vi "Configure Trigger.vi"(8 "error in":errorcluster, 11 "DAQmx Base CFG in":refnum<class "DAQmx Base CFG.lvclass">) -> (0 "error out":errorcluster, 3 "DAQmx Base CFG out":refnum<class "DAQmx Base CFG.lvclass">)   [LabVIEW 2024, in "DAQmx Base CFG.lvclass"]
uses:
  DAQmx Base CFG.lvclass
  Configurations/CFG Base/CFG Base.lvclass/CFG Base.ctl
  <vilib>/JDP Science/JSONtext/Find Item.vi
  <vilib>/JDP Science/JSONtext/Next JSON Value.vi
  <vilib>/JDP Science/JSONtext/String Subset.vi
  <vilib>/JDP Science/JSONtext/Parsing/Advance past next JSON Value (inlined COPY).vi
  <vilib>/JDP Science/JSONtext/Parsing/Advance past whitespace.vi
  <vilib>/JDP Science/JSONtext/Parsing/Advance past String.vi
  <vilib>/JDP Science/JSONtext/Parsing/Advance past Number.vi
  <vilib>/JDP Science/JSONtext/Parsing/Advance past Line Ending.vi
  <vilib>/JDP Science/JSONtext/Parsing/Parse Full Path or Item Name.vi
  <vilib>/JDP Science/JSONtext/Parsing/Advance past Array.vi
  <vilib>/JDP Science/JSONtext/Parsing/Advance past Object.vi
  <vilib>/JDP Science/JSONtext/support/Error Cluster From Code.vi
  <vilib>/JDP Science/JSONtext/Offset/Find Item Locations by Path.vi
  <vilib>/JDP Science/JSONtext/JSON text to Variant.vi
  <vilib>/JDP Science/JSONtext/LVClass Serializer/JSONtext LVClass Serializer.lvclass
  DAQmx Base CFG.lvclass/DAQmx Base CFG.ctl
  D:/git/HAL/HAL/Configurations/CFG JSON/CFG JSON.lvclass
  D:/git/HAL/HAL/Configurations/CFG Base/CFG Base.lvclass
  D:/git/HAL/HAL/Devices/DAQmx/DAQmx Base CFG/DAQmx Base CFG.lvclass
  Configurations/CFG JSON/CFG JSON.lvclass
  Configurations/CFG Base/CFG Base.lvclass
  d79926cf-9685-4438-8037-da5245ed871f.vi
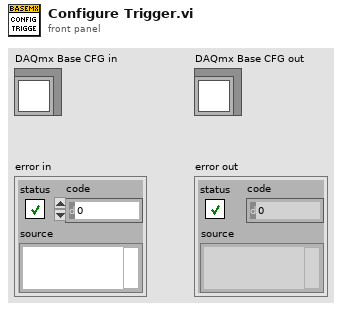
[diagram p1: front panel]
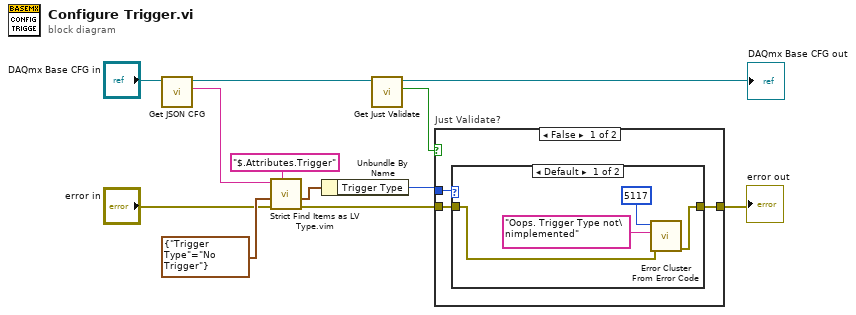
[diagram p0: block diagram]
diagram:
  n1 = call "Get JSON CFG.vi"("CFG JSON in"="DAQmx Base CFG in") -> ("<JSON> CFG"=w12:string, "CFG JSON out"=w2:refnum<class "DAQmx Base CFG.lvclass">)  [unwired: 9 in]
  n2 = call "Strict Find Items as LV Type.vim"("$Path or Item Name"="$.Attributes.Trigger", "error in"="error in", "Data Type and Default Value"=cluster{"Trigger Type":enum16{"No Trigger"}} {"Trigger Type"=enum."No Trigger"}, "<JSON>"=w12) -> ("error out"=w1:errorcluster, "Data out"=w9:cluster{"Trigger Type":enum16{"No Trigger"}})  [unwired: 5 in, 1 out]
  n3 = Unbundle By Name(w9) -> ("Trigger Type"=w8:enum16{"No Trigger"})
  n4 = call "Get Just Validate.vi"("CFG Base in"=w2) -> ("Just Validate"=w5:bool, "CFG Base out"=→"DAQmx Base CFG out":refnum<class "DAQmx Base CFG.lvclass">)  [unwired: 9 in]
  n5 = case "Just Validate?" shown="False" w5 {
    tunnel: w8 -> [w15 _]
    tunnel: w1 -> [w14 w21]
    tunnel: [w13 w21] -> w7
    frame False {
      n6 = case shown="Default" w15 {
        tunnel: w14 -> [w16 w20]
        tunnel: [w19 w20] -> w13
        frame Default {
          n7 = call <vilib>:"Error Cluster From Error Code.vi"("error in (no error)"=w16, "error message (\"\")"="Oops. Trigger Type not\nimplemented" ("error message (\"\")"), "error code (0)"=5117) -> ("error out"=w19:errorcluster)  [unwired: 6 in]
        }
        frame "No Trigger" {
        }
      }
    }
    frame True {
    }
  }
  "error out" <- w7
